vi "Configure Clock.vi"(8 "error in (no error)":errorcluster, 10 "samples per channel":i32=1000, 11 "NIDIO in":refnum<class "NIDIO.lvclass">) -> (0 "error out":errorcluster, 3 "NIDIO out":refnum<class "NIDIO.lvclass">)   [LabVIEW 2015, in "NIDIO.lvclass"]
uses:
  NIDIO.lvclass
  NIDIO.lvclass/NIDIO.ctl
  <vilib>/DAQmx/configure/timing.llb/DAQmx Timing (Sample Clock).vi
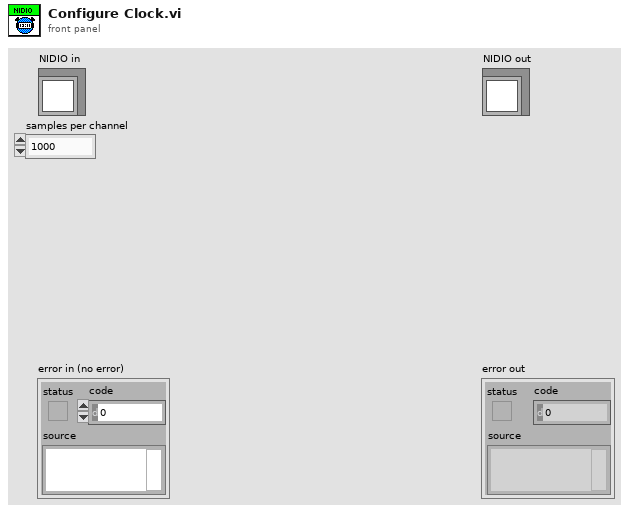
[diagram p1: front panel]
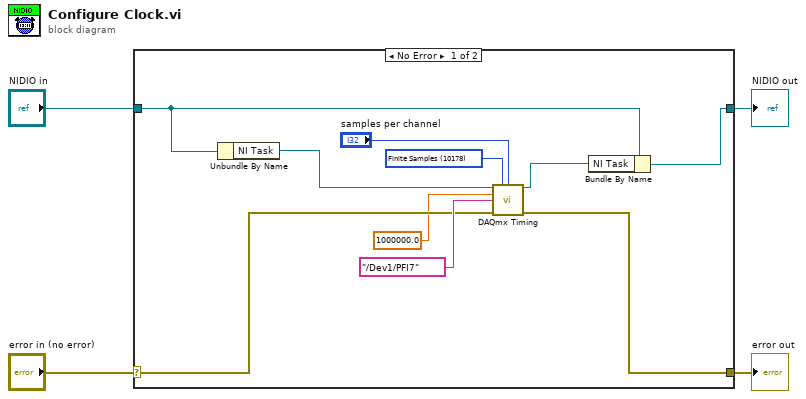
[diagram p0: block diagram]
diagram:
  n1 = case shown="No Error" "error in (no error)" {
    selector: "error in (no error)" -> [w10 w16]
    tunnel: [w9 w16] -> w3
    tunnel: [w6 w15] -> w1
    tunnel: "NIDIO in" -> [w8 w15]
    frame No Error {
      w13 = 10178 items=["Finite Samples"=10178, "Continuous Samples"=10123, "Hardware Timed Single Point"=12522] ("sample mode")
      n2 = Unbundle By Name(w8) -> ("NI Task"=w12:refnum<k21>)
      n3 = call-poly <vilib>:"DAQmx Timing.vi"("task/channels in"=w12, "sample mode"=w13, "samples per channel"="samples per channel", "rate"=1000000.0, "source"=tag "/Dev1/PFI7", "error in"=w10) -> ("task out"=w7:refnum<k21>, "error out"=w9:errorcluster)  [unwired: 8 in]
      n4 = Bundle By Name(cluster=w8, "NI Task"=w7) -> (w6:refnum<class "NIDIO.lvclass">)
    }
    frame Error {
    }
  }
  "error out" <- w3
  "NIDIO out" <- w1
